vi "sv_Autoscale for Octave.vi"(1 "scale":cluster{"min":dbl, "max":dbl} {"max" format="%.2f"; "min" format="%.2f"}) -> (0 "autoscale":cluster{"min":dbl, "max":dbl} {"max" format="%.2f"; "min" format="%.2f"})   [LabVIEW 2017]
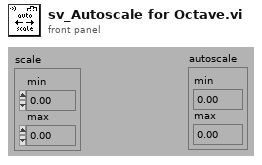
[diagram p1: front panel]
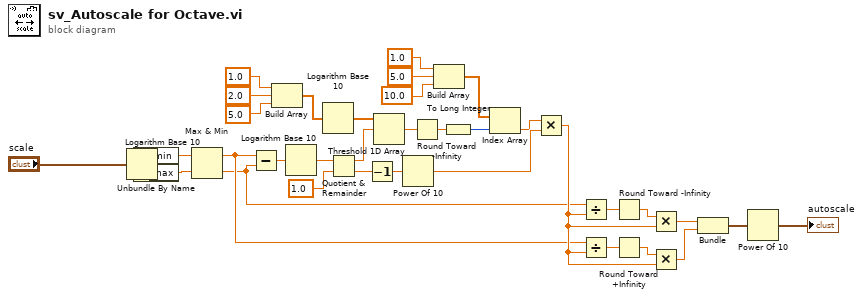
[diagram p0: block diagram]
diagram:
  n1 = Logarithm Base 10(1:"scale") -> (0:w2:cluster{"min":dbl, "max":dbl})
  n2 = Unbundle By Name(w2) -> ("min"=w4:dbl, "max"=w3:dbl)
  n3 = Max & Min(x=w4, y=w3) -> (max(x,y)=w6:dbl, min(x,y)=w5:dbl)
  n4 = Subtract(x=w6, y=w5) -> (x-y=w34:dbl)
  n5 = Build Array(1.0 ("x"), 2.0 ("x"), 5.0 ("x")) -> (w12:dbl[])
  n6 = Logarithm Base 10(1:w34) -> (0:w31:dbl)
  n7 = Logarithm Base 10(1:w12) -> (0:w28:dbl[])
  n8 = Quotient & Remainder(x=w31, y=1.0) -> (x-y*floor(x/y)=w27:dbl, floor(x/y)=w25:dbl)
  n9 = Decrement(x=w25) -> (x-1=w24:dbl)
  n10 = Threshold 1D Array(2:w27, 3:w28) -> (0:w23:dbl)  [unwired: 1 in]
  n11 = Power Of 10(x=w24) -> (10^x=w20:dbl)
  n12 = Round Toward -Infinity(1:w23) -> (0:w22:dbl)
  n13 = Build Array(1.0 ("x"), 5.0 ("x"), 10.0 ("x")) -> (w9:dbl[])
  n14 = To Long Integer(number=w22) -> (32bit integer=w21:i32)
  n15 = Index Array(array=w9, index=w21) -> (element=w19:dbl)
  n16 = Multiply(x=w19, y=w20) -> (x*y=w16:dbl)
  n17 = Divide(x=w5, y=w16) -> (x/y=w17:dbl)
  n18 = Divide(x=w6, y=w16) -> (x/y=w33:dbl)
  n19 = Round Toward -Infinity(1:w17) -> (0:w18:dbl)
  n20 = Round Toward +Infinity(x=w33) -> (ceil(x): smallest int >= x=w32:dbl)
  n21 = Multiply(x=w18, y=w16) -> (x*y=w15:dbl)
  n22 = Multiply(x=w32, y=w16) -> (x*y=w14:dbl)
  n23 = Bundle(w15, w14) -> (w13:cluster{dbl, dbl})  [unwired: 1 in]
  n24 = Power Of 10(x=w13) -> (10^x=→"autoscale":cluster{dbl, dbl})
